vi "Configure.vi"(8 "error in (no error)":errorcluster, 9 "Path":path, 10 "Interactive?":bool, 11 "Report Interface in":refnum<class "Report Plugin.lvclass">) -> (0 "error out":errorcluster, 3 "Report Interface out":refnum<class "Report Plugin.lvclass">)   [LabVIEW 2020, in "Report Plugin.lvclass"]
doc: "This method is called by the framework when the user selects the configure option in the reoport configuration dialog. It is also called by the framework when the plugin is initized to load the configurations from disk. \nThe implementation shall have two modes selected by the interactive? control. If in interactive, the VI should provide the user with a configuration window to edit the settings of the plugin.\nWhen interactive is set to false, the settngs should be loaded from disk and a configured object passed out. \nIf there is a file path provided to the Path input, this must be used over the value read from disk. This is used by the API to control where reports are stored and should not rely on configurations or system settings"
uses:
  Report Plugin.lvclass
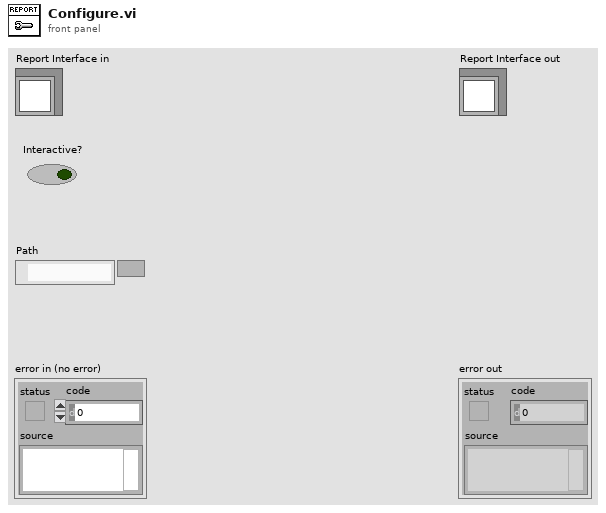
[diagram p1: front panel]
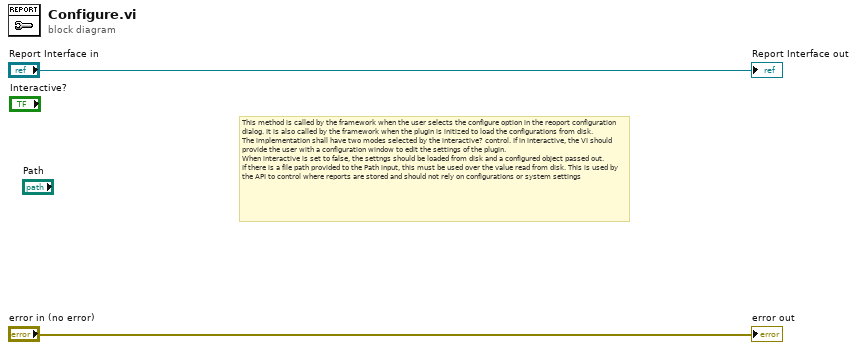
[diagram p0: block diagram]
diagram:
  # "This method is called by the framework when the user selects the configure option in the reoport configuration dialog. It is also called by the framework when the plugin is initized to load the configurations from disk. \nThe implementation shall have two modes selected by the interactive? control. If in interactive, the VI should provide the user with a configuration window to edit the settings of the plugin.\nWhen interactive is set to false, the settngs should be loaded from disk and a configured object passed out. \nIf there is a file path provided to the Path input, this must be used over the value read from disk. This is used by the API to control where reports are stored and should not rely on configurations or system settings"
  "error out" <- "error in (no error)"
  "Report Interface out" <- "Report Interface in"
